vi "质量信息录入.vi"(0 "检测项目":string, 1 "功能":enum16{"录入", "清空"}(ring), 5 "单位":string, 7 "检测值":string, 9 "检测结果":bool, 11 "错误输入（无错误）":errorcluster, 12 "标准值":string) -> (15 "错误输出":errorcluster)   [LabVIEW 2017]
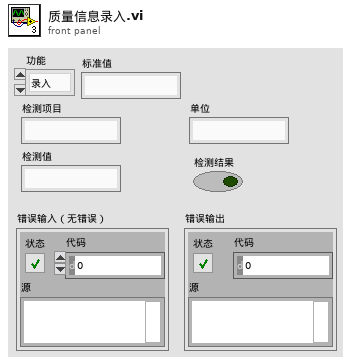
[diagram p1: front panel]
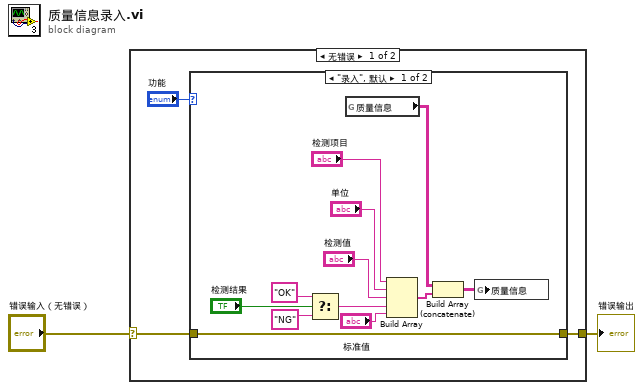
[diagram p0: block diagram]
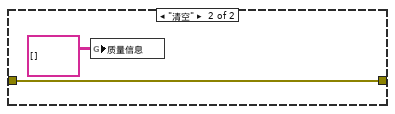
[diagram p2: hidden frame]
diagram:
  n1 = case shown="无错误" "错误输入（无错误）" {
    selector: "错误输入（无错误）" -> [w4 w20]
    tunnel: [w3 w20] -> w1
    frame No Error {
      n2 = case shown="\"录入\", 默认" "功能" {
        tunnel: [w7 w18] -> w3
        tunnel: w4 -> [w7 w18]
        frame "录入", Default {
          n3 = Select(t="OK", s="检测结果", f="NG") -> (s? t:f=w12:string)
          n4 = global read "追溯全部变量.vi" "质量信息"() -> (w9:string[][])
          n5 = Build Array("检测项目", "单位", "检测值", w12, "标准值") -> (w10:string[])
          n6 = Build Array (concatenate)(w9, w10) -> (w8:string[][])
          n7 = global write "追溯全部变量.vi" "质量信息"(w8) -> ()
        }
        frame "清空" {
          n8 = global write "追溯全部变量.vi" "质量信息"(string[][] [] ("物料信息")) -> ()
        }
      }
    }
    frame Error {
    }
  }
  "错误输出" <- w1
